vi "Save.vi"(8 "error in (no error)":errorcluster) -> (0 "error out":errorcluster)   [LabVIEW 2018]
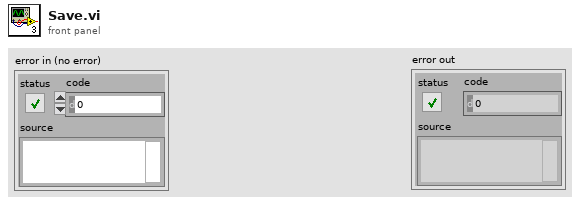
[diagram p1: front panel]
types:
  T1 = enum16{"open", "replace", "create", "open or create", "replace or create", "replace or create with confirmation"}
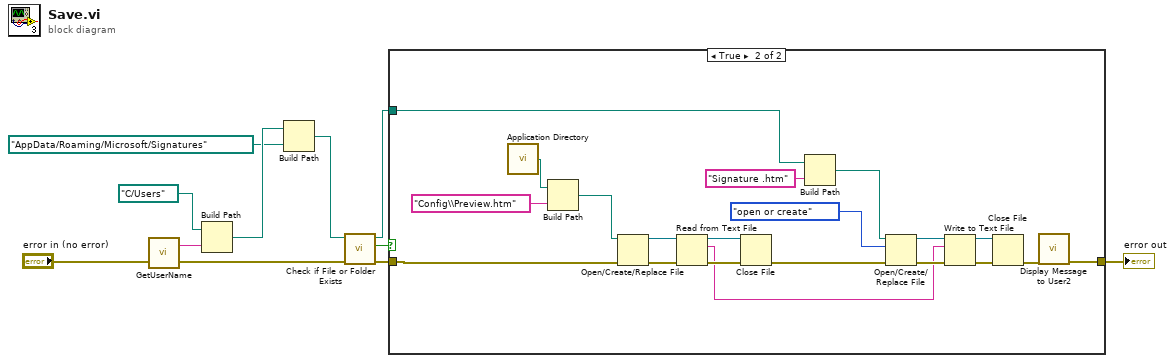
[diagram p0: block diagram]
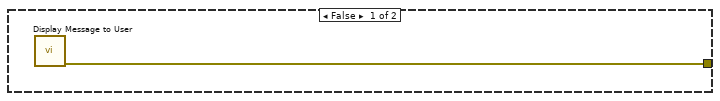
[diagram p2: hidden frame]
diagram:
  n1 = call "GetUserName.vi"("error in (no error)"="error in (no error)") -> ("error out"=w6:errorcluster, "User Name"=w9:string)  [unwired: 1 in]
  n2 = Build Path(base path=path "C:/Users" ("path"), name or relative path=w9) -> (appended path=w8:path)
  n3 = Build Path(base path=w8, name or relative path=path "AppData/Roaming/Microsoft/Signatures" ("path")) -> (appended path=w5:path)
  n4 = call <vilib>:"Check if File or Folder Exists.vi"("error in (no error)"=w6, "path"=w5) -> ("error out"=w3:errorcluster, "file or folder exists?"=w4:bool, "dup path"=w2:path)  [unwired: 7 in]
  n5 = case shown="True" w4 {
    tunnel: w3 -> [_ w30]
    tunnel: w2 -> [_ w24]
    tunnel: [w12 w14] -> w1
    frame False {
      n6 = call "Display Message to User"() -> ("error out"=w12:errorcluster)  [unwired: 10 in, 1 out]
    }
    frame True {
      n7 = call <vilib>:"Application Directory.vi"() -> ("Application Directory"=w32:path)
      n8 = Build Path(base path=w32, name or relative path="Config\\Preview.htm") -> (appended path=w29:path)
      n9 = Open/Create/Replace File(file path (use dialog)=w29, error in=w30) -> (refnum out=w27:refnum<file>, error out=w28:errorcluster)  [unwired: 4 in, 1 out]
      n10 = Read from Text File(file (use dialog)=w27, error in=w28) -> (refnum out=w25:refnum<file>, text=w15:string, error out=w26:errorcluster)  [unwired: 2 in, 1 out]
      n11 = Close File(refnum=w25, error in=w26) -> (error out=w20:errorcluster)  [unwired: 1 out]
      n12 = Build Path(base path=w24, name or relative path="Signature .htm") -> (appended path=w19:path)
      n13 = Open/Create/Replace File(file path (use dialog)=w19, error in=w20, operation (0:open)=T1."open or create") -> (refnum out=w21:refnum<file>, error out=w18:errorcluster)  [unwired: 3 in, 1 out]
      n14 = Write to Text File(file (use dialog)=w21, text=w15, error in=w18) -> (refnum out=w22:refnum<file>, error out=w17:errorcluster)  [unwired: 1 in, 1 out]
      n15 = Close File(refnum=w22, error in=w17) -> (error out=w13:errorcluster)  [unwired: 1 out]
      n16 = call "Display Message to User2"("error in (no error)"=w13) -> ("error out"=w14:errorcluster)  [unwired: 9 in, 1 out]
    }
  }
  "error out" <- w1
